vi "PPFS_DRIVE_BEGIN.vi"(8 "error in (no error)":errorcluster) -> (0 "error out":errorcluster, 2 "Gyro Reading":T1 {"SIN" format="%13.4f"; "COS" format="%13.4f"; "VALUE" format="%13.4f"}, 3 "SWERVE_DRIVE_KINEMATICS":T2 {"SavedModuleStates"."Angle"."SIN" format="%13.4f"; "SavedModuleStates"."Angle"."COS" format="%13.4f"; "SavedModuleStates"."Angle"."VALUE" format="%13.4f"; "PrevCoR"."Y" format="%14.3f"; "PrevCoR"."X" format="%14.3f"; "Modules"."Y" format="%14.3f"; "Modules"."X" format="%14.3f"})   [LabVIEW 2023]
uses:
  <vilib>/Rock Robotics/WPI/ThirdParty/JAS_Junk/TrajLib/TypeDef/SWERVE_DRIVE_KINEMATICS.ctl
  <vilib>/Analysis/Matrix/Datatypes/RealMatrix.ctl
  <vilib>/Rock Robotics/WPI/ThirdParty/JAS_Junk/TrajLib/TypeDef/TRANSLATION2D.ctl
  <vilib>/Rock Robotics/WPI/ThirdParty/JAS_Junk/TrajLib/TypeDef/SWERVE_DRIVE_MODULE_STATE.ctl
  <vilib>/Rock Robotics/WPI/ThirdParty/JAS_Junk/TrajLib/TypeDef/ROTATION2D.ctl
  <vilib>/Rock Robotics/WPI/ThirdParty/JAS_Junk/TrajLib/Conv_Deg_Radians.vi
  <vilib>/Rock Robotics/WPI/ThirdParty/JAS_Junk/TrajLib/Rotation2d_CreateAngle.vi
  <vilib>/Rock Robotics/WPI/ThirdParty/JAS_Junk/TrajLib/VI/BoolCmd_Send_Internal.vi
  <vilib>/Rock Robotics/WPI/ThirdParty/JAS_Junk/TrajLib/VI/BoolCmd_ObtainQueue.vi
  PPFS_DRIVE_GLOBALS.vi
  <vilib>/Rock Robotics/WPI/ThirdParty/JAS_Junk/TrajLib/Trajectory_Library.lvlib
  <vilib>/Analysis/Matrix/NI_Matrix.lvlib
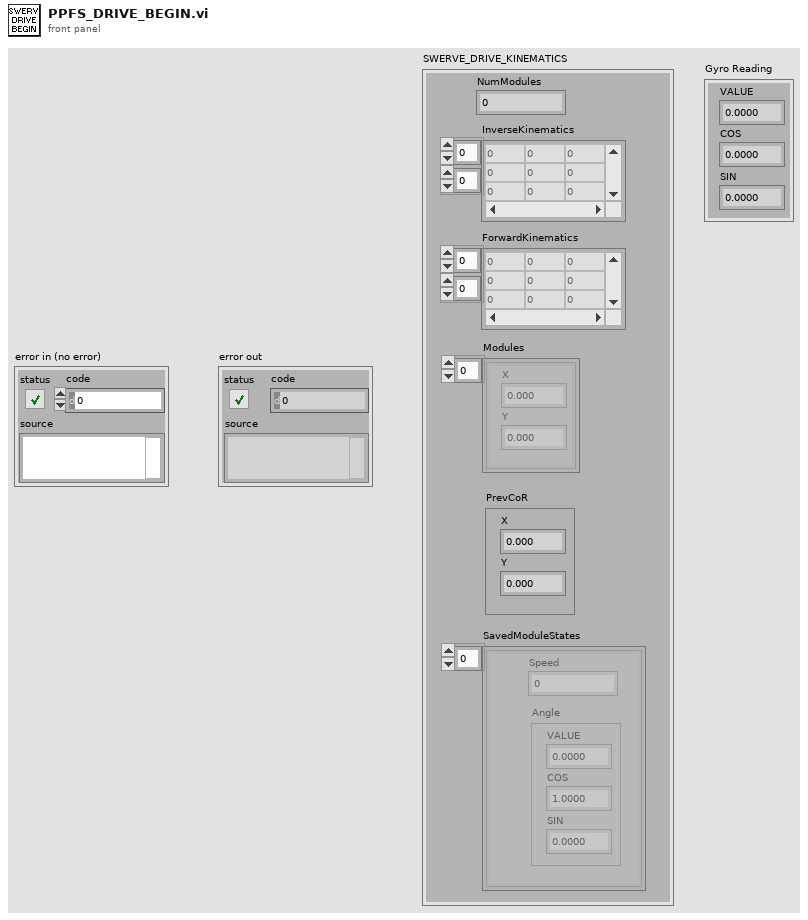
[diagram p1: front panel]
types:
  T1 = typedef "Trajectory_Library.lvlib/ROTATION2D.ctl" = cluster{"VALUE":dbl, "COS":dbl, "SIN":dbl}
  T2 = typedef "Trajectory_Library.lvlib/SWERVE_DRIVE_KINEMATICS.ctl" = cluster{"NumModules":i32, "InverseKinematics":T3, "ForwardKinematics":T3, "Modules":T4[], "PrevCoR":T4, "SavedModuleStates":T5[]}
  T3 = typedef "NI_Matrix.lvlib/RealMatrix.ctl" = dbl[][]
  T4 = typedef "Trajectory_Library.lvlib/TRANSLATION2D.ctl" = cluster{"X":dbl, "Y":dbl}
  T5 = typedef "Trajectory_Library.lvlib/SWERVE_DRIVE_MODULE_STATE.ctl" = cluster{"Speed":dbl, "Angle":T1}
  T6 = typedef "Trajectory_Library.lvlib/SWERVE_DRIVE_MODULE_POSITION.ctl" = cluster{"Distance":dbl, "Angle":T1, "P":bool}
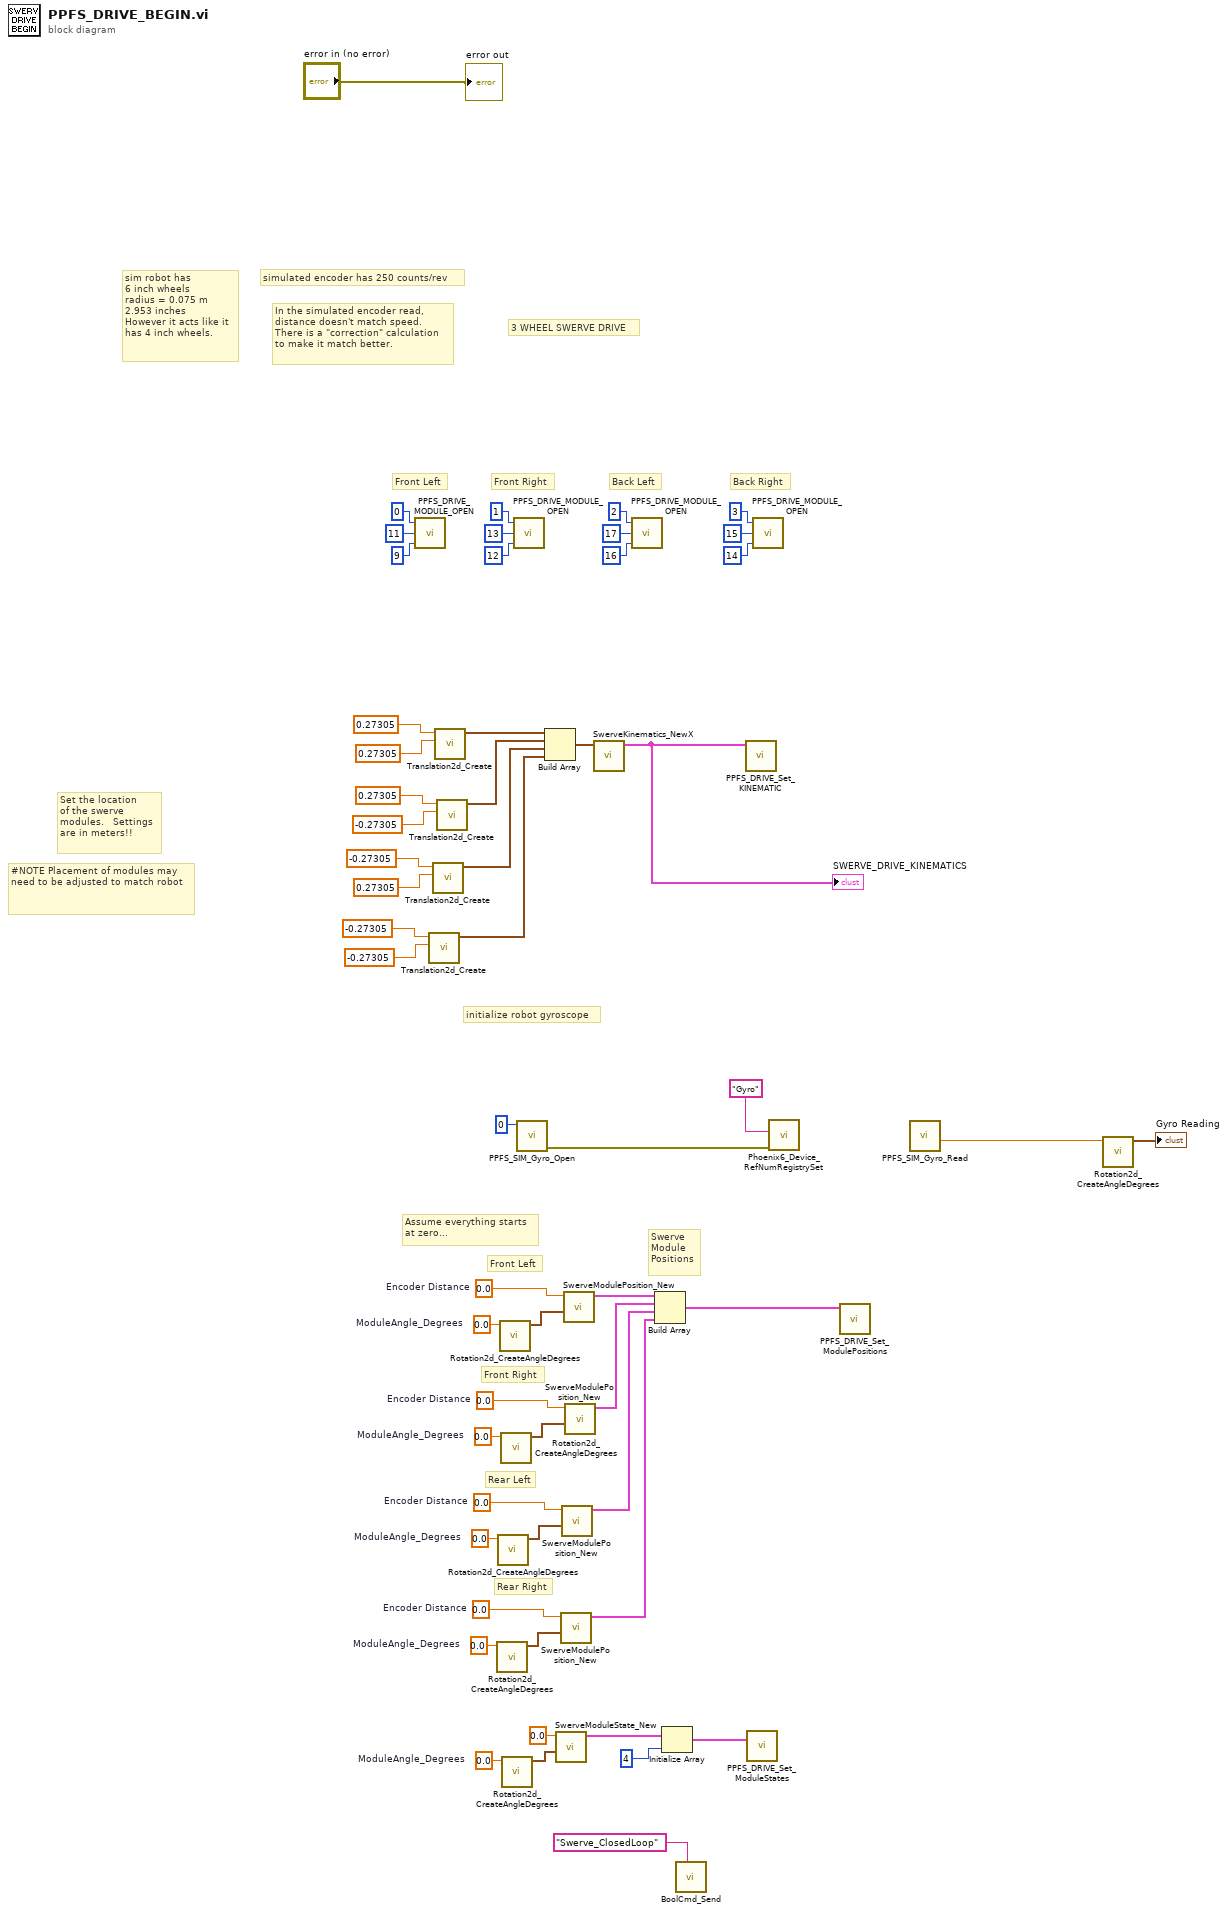
[diagram p0: block diagram]
diagram:
  w19 = 0.0  # ModuleAngle_Degrees
  w38 = 0.0  # ModuleAngle_Degrees
  w36 = 0.0  # Encoder Distance
  w35 = 0.0  # ModuleAngle_Degrees
  w33 = 0.0  # Encoder Distance
  w32 = 0.0  # ModuleAngle_Degrees
  w30 = 0.0  # Encoder Distance
  w28 = 0.0  # ModuleAngle_Degrees
  w26 = 0.0  # Encoder Distance
  # "Back Right"
  # "Back Left"
  # "Front Right"
  # "Front Left"
  # "Assume everything starts\nat zero..."
  # "Front Left"
  # "Swerve\nModule\nPositions"
  # "Rear Right"
  # "Rear Left"
  # "Front Right"
  # "#NOTE Placement of modules may need to be adjusted to match robot"
  # "Set the location\nof the swerve \nmodules.   Settings\nare in meters!!"
  # "3 WHEEL SWERVE DRIVE"
  # "initialize robot gyroscope"
  # "In the simulated encoder read,\ndistance doesn't match speed.\nThere is a \"correction\" calculation\nto make it match better."
  # "simulated encoder has 250 counts/rev"
  # "sim robot has\n6 inch wheels\nradius = 0.075 m\n2.953 inches\nHowever it acts like it\nhas 4 inch wheels."
  n1 = call "PPFS_DRIVE_MODULE_OPEN.vi"("Swerve CAN ID"=u8 9, "Drive CAN ID"=u8 11, "Module Index"=0 ("NameSuffix")) -> ()  [unwired: 1 in]
  n2 = call <vilib>:"Translation2d_Create.vi"("Y"=-0.27305, "X"=-0.27305) -> ("TRANSLATION"=w56:T4)  [unwired: 9 in]
  n3 = call <vilib>:"Translation2d_Create.vi"("Y"=0.27305, "X"=-0.27305) -> ("TRANSLATION"=w52:T4)  [unwired: 9 in]
  n4 = call <vilib>:"Translation2d_Create.vi"("Y"=0.27305, "X"=0.27305) -> ("TRANSLATION"=w50:T4)  [unwired: 9 in]
  n5 = call <vilib>:"Translation2d_Create.vi"("Y"=-0.27305, "X"=0.27305) -> ("TRANSLATION"=w51:T4)  [unwired: 9 in]
  n6 = call <vilib>:"Rotation2d_CreateAngleDegrees.vi"("Angle_Degrees"=w38) -> ("ROTATION"=w37:T1)  [unwired: 10 in]
  n7 = call <vilib>:"Rotation2d_CreateAngleDegrees.vi"("Angle_Degrees"=w35) -> ("ROTATION"=w34:T1)  [unwired: 10 in]
  n8 = call <vilib>:"Rotation2d_CreateAngleDegrees.vi"("Angle_Degrees"=w28) -> ("ROTATION"=w27:T1)  [unwired: 10 in]
  n9 = call <vilib>:"Rotation2d_CreateAngleDegrees.vi"("Angle_Degrees"=w32) -> ("ROTATION"=w31:T1)  [unwired: 10 in]
  n10 = call <vilib>:"Rotation2d_CreateAngleDegrees.vi"("Angle_Degrees"=w19) -> ("ROTATION"=w18:T1)  [unwired: 10 in]
  n11 = call "PPFS_DRIVE_MODULE_OPEN.vi"("Swerve CAN ID"=u8 12, "Drive CAN ID"=u8 13, "Module Index"=1 ("NameSuffix")) -> ()  [unwired: 1 in]
  n12 = call "PPFS_SIM_Gyro_Open.vi"("IMU CAN ID"=u8 0) -> ("error out"=w24:errorcluster)  [unwired: 6 in, 1 out]
  n13 = Build Array(w50, w51, w52, w56) -> (w53:T4[])
  n14 = call <vilib>:"SwerveModuleState_New.vi"("ROTATION"=w18, "Speed"=0.0) -> ("SWERVE_DRIVE_MODULE_STATE"=w17:T5)  [unwired: 9 in]
  n15 = call <vilib>:"SwerveModulePosition_New.vi"("ROTATION"=w37, "Distance"=w36) -> ("SWERVE_DRIVE_MODULE_POSITION"=w41:T6)  [unwired: 9 in]
  n16 = call <vilib>:"SwerveModulePosition_New.vi"("ROTATION"=w34, "Distance"=w33) -> ("SWERVE_DRIVE_MODULE_POSITION"=w40:T6)  [unwired: 9 in]
  n17 = call <vilib>:"SwerveModulePosition_New.vi"("ROTATION"=w27, "Distance"=w26) -> ("SWERVE_DRIVE_MODULE_POSITION"=w29:T6)  [unwired: 9 in]
  n18 = call <vilib>:"SwerveModulePosition_New.vi"("ROTATION"=w31, "Distance"=w30) -> ("SWERVE_DRIVE_MODULE_POSITION"=w39:T6)  [unwired: 9 in]
  n19 = call <vilib>:"SwerveKinematics_NewX.vi"("Wheels"=w53) -> ("SWERVE_DRIVE_KINEMATICS"=w15:T2)  [unwired: 10 in]
  "SWERVE_DRIVE_KINEMATICS" <- w15
  n20 = call "PPFS_DRIVE_MODULE_OPEN.vi"("Swerve CAN ID"=u8 16, "Drive CAN ID"=u8 17, "Module Index"=2 ("NameSuffix")) -> ()  [unwired: 1 in]
  n21 = Build Array(w29, w39, w40, w41) -> (w16:T6[])
  n22 = Initialize Array(w17, 4 ("dimension size")) -> (w14:T5[])
  n23 = call <vilib>:"BoolCmd_Send.vi"("Command Name"="Swerve_ClosedLoop") -> ()  [unwired: 10 in, 1 out]
  n24 = call "PPFS_DRIVE_Set_KINEMATIC.vi"("SWERVE_DRIVE_KINEMATICS"=w15) -> ()  [unwired: 11 in]
  n25 = call "PPFS_DRIVE_Set_ModuleStates.vi"("Swerve Module States"=w14) -> ()  [unwired: 11 in]
  n26 = call "PPFS_DRIVE_MODULE_OPEN.vi"("Swerve CAN ID"=u8 14, "Drive CAN ID"=u8 15, "Module Index"=3 ("NameSuffix")) -> ()  [unwired: 1 in]
  n27 = call <vilib>:"Phoenix6_Device_RefNumRegistrySet.vi"("error in (no error)"=w24, "refnum name"="Gyro") -> ()  [unwired: 8 in, 2 out]
  n28 = call "PPFS_DRIVE_Set_ModulePositions.vi"("Swerve Module Positions"=w16) -> ()  [unwired: 11 in]
  n29 = call "PPFS_SIM_Gyro_Read.vi"() -> ("Gyro_Cont_Deg"=w23:dbl)  [unwired: 11 in]
  n30 = call <vilib>:"Rotation2d_CreateAngleDegrees.vi"("Angle_Degrees"=w23) -> ("ROTATION"=→"Gyro Reading":T1)  [unwired: 10 in]
  "error out" <- "error in (no error)"
